vi "Clusterwitharraymenuring.vi"(1 "Cluster In":cluster{"Array In":u16[], "Ring":u16} {"Ring" items=["A", "B", "C"]; "Array In" items=["A", "B", "C"]}) -> (0 "Cluster Out":cluster{"Array Out":u16[], "Ring":u16} {"Ring" items=["A", "B", "C"]; "Array Out" items=["A", "B", "C"]})   [LabVIEW 2011]
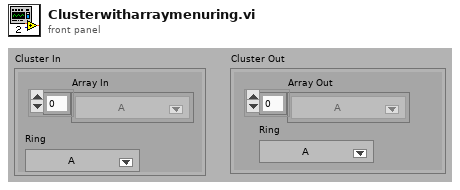
[diagram p1: front panel]
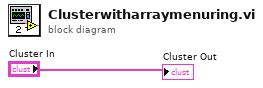
[diagram p0: block diagram]
diagram:
  "Cluster Out" <- "Cluster In"
